vi "关键参数交互.vi"(9 "量程下拉列表":refnum<vi>, 10 "测量模式下拉列表":refnum<vi>, 11 "参数下拉列表":refnum<vi>) -> ()   [LabVIEW 2016]
panel:
  out "x != y? 2":T1
  out "x != y?":T1
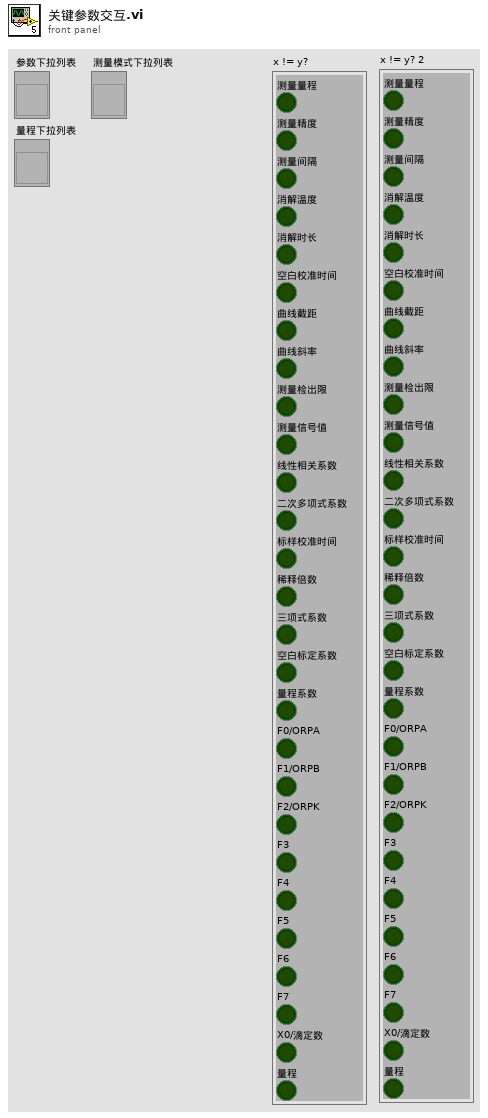
[diagram p1: front panel]
types:
  T1 = cluster{"测量量程":bool, "测量精度":bool, "测量间隔":bool, "消解温度":bool, "消解时长":bool, "空白校准时间":bool, "曲线截距":bool, "曲线斜率":bool, "测量检出限":bool, "测量信号值":bool, "线性相关系数":bool, "二次多项式系数":bool, "标样校准时间":bool, "稀释倍数":bool, "三项式系数":bool, "空白标定系数":bool, "量程系数":bool, "F0/ORPA":bool, "F1/ORPB":bool, "F2/ORPK":bool, "F3":bool, "F4":bool, "F5":bool, "F6":bool, "F7":bool, "X0/滴定数":bool, "量程":bool}
  T2 = cluster{"chose":string, "公式":cluster{"X^2":dbl, "X":dbl, "b":dbl}}
  T3 = cluster{"测量量程":dbl, "测量精度":dbl, "测量间隔":dbl, "消解温度":dbl, "消解时长":dbl, "空白校准时间":timestamp, "曲线截距":dbl, "曲线斜率":dbl, "测量检出限":dbl, "测量信号值":dbl, "线性相关系数":dbl, "二次多项式系数":dbl, "标样校准时间":timestamp, "稀释倍数":dbl, "三项式系数":dbl, "空白标定系数":dbl, "量程系数":dbl, "F0/ORPA":dbl, "F1/ORPB":dbl, "F2/ORPK":dbl, "F3":dbl, "F4":dbl, "F5":dbl, "F6":dbl, "F7":dbl, "X0/滴定数":dbl, "量程":dbl}
  T4 = cluster{"时间标识":timestamp, "设备":string, "日志信息":string, "流程参数":string}
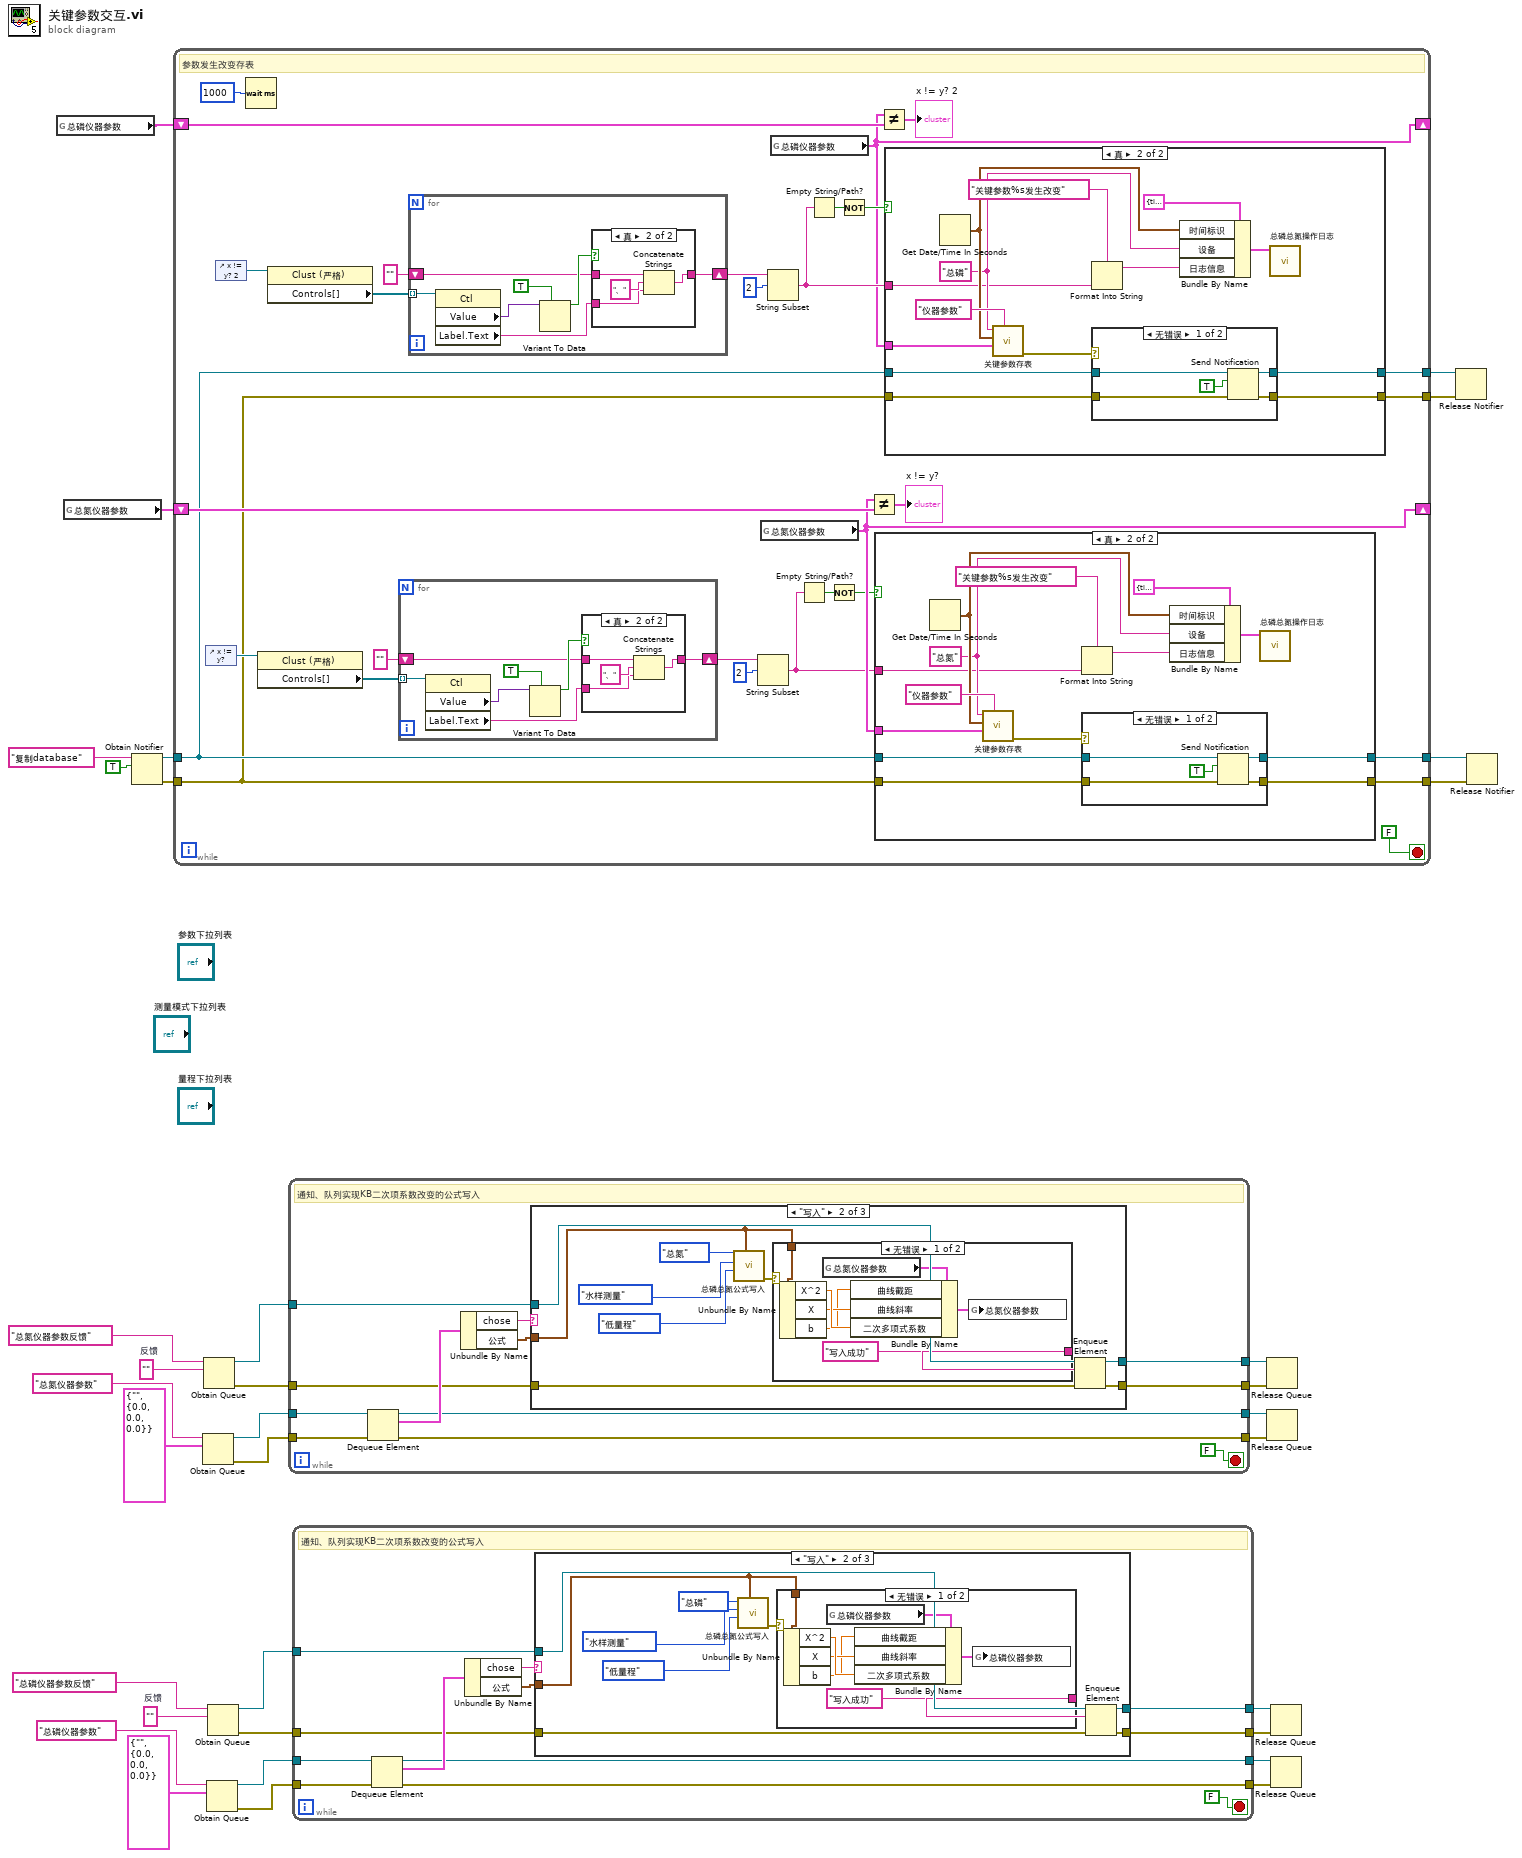
[diagram p0: block diagram]
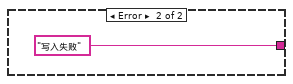
[diagram p3: hidden frame]
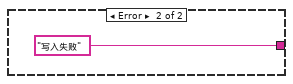
[diagram p6: hidden frame]
diagram:
  w10 = ""  # 反馈
  w27 = ""  # 反馈
  n1 = global read "总磷总氮断电保存全局变量.vi" "总磷仪器参数"() -> (w3:T3)
  n2 = global read "总磷总氮断电保存全局变量.vi" "总氮仪器参数"() -> (w34:T3)
  n3 = Obtain Notifier(name (unnamed)="复制database" ("名称（未命名）"), notification data type=TRUE) -> (notifier out=w19:refnum<notifier>, error out=w18:errorcluster)  [unwired: 2 in, 1 out]
  n4 = while {
    shift-right: [w59] -> _
    shift-left: w34 -> [w62]
    tunnel: w19 -> [w38]
    tunnel: w18 -> [w37]
    tunnel: [w58] -> w17
    tunnel: [w57] -> w16
    shift-right: [w39] -> _
    shift-left: w3 -> [w40]
    tunnel: [w36] -> w2
    tunnel: [w35] -> w1
    stop <- FALSE stop-if-true
    # "参数发生改变存表"
    n5 = control-ref of="x != y?"() -> (w60:refnum<vi>)
    n6 = control-ref of="x != y? 2"() -> (w42:refnum<vi>)
    n7 = Wait (ms)(milliseconds to wait=u32 1000 ("等待时间（毫秒）")) -> ()  [unwired: 1 out]
    n8 = property class="Clust (严格)"(reference=w60) -> ("Controls[]"=w53:refnum<vi>[])  [unwired: 1 in, 2 out]
    n9 = property class="Clust (严格)"(reference=w42) -> ("Controls[]"=w46:refnum<vi>[])  [unwired: 1 in, 2 out]
    n10 = for {
      tunnel: w53 -> [w106] mode=indexing
      shift-right: [w100] -> w55
      shift-left: "" -> [w102]
      n11 = property class="Ctl"(reference=w106) -> ("Value"=w104:variant, "Label.Text"=w101:string)  [unwired: 1 in, 2 out]
      n12 = Variant To Data(type=TRUE, Variant=w104) -> (data=w103:bool)  [unwired: 1 in, 1 out]
      n13 = case shown="真" w103 {
        tunnel: w102 -> [w107 w111]
        tunnel: w101 -> [_ w108]
        tunnel: [w107 w110] -> w100
        frame False {
        }
        frame True {
          n14 = Concatenate Strings(w111, "、", w108) -> (w110:string)
        }
      }
    }
    n15 = for {
      tunnel: w46 -> [w71] mode=indexing
      shift-right: [w65] -> w44
      shift-left: "" -> [w67]
      n16 = property class="Ctl"(reference=w71) -> ("Value"=w69:variant, "Label.Text"=w66:string)  [unwired: 1 in, 2 out]
      n17 = Variant To Data(type=TRUE, Variant=w69) -> (data=w68:bool)  [unwired: 1 in, 1 out]
      n18 = case shown="真" w68 {
        tunnel: w67 -> [w72 w76]
        tunnel: w66 -> [_ w73]
        tunnel: [w72 w75] -> w65
        frame False {
        }
        frame True {
          n19 = Concatenate Strings(w76, "、", w73) -> (w75:string)
        }
      }
    }
    n20 = String Subset(string=w55, offset (0)=2 ("偏移量(0)")) -> (substring=w50:string)  [unwired: 1 in]
    n21 = global read "总磷总氮断电保存全局变量.vi" "总氮仪器参数"() -> (w59:T3)
    n22 = String Subset(string=w44, offset (0)=2 ("偏移量(0)")) -> (substring=w49:string)  [unwired: 1 in]
    n23 = global read "总磷总氮断电保存全局变量.vi" "总磷仪器参数"() -> (w39:T3)
    n24 = Empty String/Path?(string/path=w50) -> (empty?=w52:bool)
    n25 = Empty String/Path?(string/path=w49) -> (empty?=w47:bool)
    n26 = Not(x=w52) -> (.not. x?=w51:bool)
    n27 = Not(x=w47) -> (.not. x?=w48:bool)
    n28 = Not Equal?(x=w59, y=w62) -> (x != y?=→"x != y?":T1)
    n29 = case shown="真" w51 {
      tunnel: w59 -> [_ w126]
      tunnel: w50 -> [_ w120]
      tunnel: w38 -> [w113 w118]
      tunnel: w37 -> [w112 w117]
      tunnel: [w113 w115] -> w58
      tunnel: [w112 w114] -> w57
      frame False {
      }
      frame True {
        w122 = "总氮" ("仪器名称")
        n30 = Get Date/Time In Seconds() -> (seconds since 1Jan1904=w123:timestamp)
        n31 = call "关键参数存表.vi"("table"="仪器参数", "仪器参数"=w126, "datatime"=w123, "仪器名称"=w122) -> ("error out"=w116:errorcluster)  [unwired: 7 in]
        n32 = Format Into String(format string="关键参数%s发生改变" ("格式字符串"), w120) -> (resulting string=w119:string)  [unwired: 2 in, 1 out]
        n33 = case shown="无错误" w116 {
          tunnel: w118 -> [w132 w134]
          tunnel: w117 -> [w131 w133]
          tunnel: [w129 w134] -> w115
          tunnel: [w128 w133] -> w114
          frame No Error {
            n34 = Send Notification(notification=TRUE ("通知"), notifier=w132, error in (no error)=w131) -> (notifier out=w129:refnum<notifier>, error out=w128:errorcluster)
          }
          frame Error {
          }
        }
        n35 = Bundle By Name(cluster=T4 {"时间标识"=timestamp(0 s since 1904-01-01), "设备"="", "日志信息"="", "流程参数"=""} ("data in"), "时间标识"=w123, "设备"=w122, "日志信息"=w119) -> (w124:T4)
        n36 = call "总磷总氮操作日志.vi"("data in"=w124) -> ()  [unwired: 11 in]
      }
    }
    n37 = Not Equal?(x=w39, y=w40) -> (x != y?=→"x != y? 2":T1)
    n38 = case shown="真" w48 {
      tunnel: w39 -> [_ w91]
      tunnel: w49 -> [_ w85]
      tunnel: w38 -> [w78 w83]
      tunnel: w37 -> [w77 w82]
      tunnel: [w78 w80] -> w36
      tunnel: [w77 w79] -> w35
      frame False {
      }
      frame True {
        w87 = "总磷" ("仪器名称")
        n39 = Get Date/Time In Seconds() -> (seconds since 1Jan1904=w88:timestamp)
        n40 = call "关键参数存表.vi"("table"="仪器参数", "仪器参数"=w91, "datatime"=w88, "仪器名称"=w87) -> ("error out"=w81:errorcluster)  [unwired: 7 in]
        n41 = Format Into String(format string="关键参数%s发生改变" ("格式字符串"), w85) -> (resulting string=w84:string)  [unwired: 2 in, 1 out]
        n42 = case shown="无错误" w81 {
          tunnel: w83 -> [w97 w99]
          tunnel: w82 -> [w96 w98]
          tunnel: [w94 w99] -> w80
          tunnel: [w93 w98] -> w79
          frame No Error {
            n43 = Send Notification(notification=TRUE ("通知"), notifier=w97, error in (no error)=w96) -> (notifier out=w94:refnum<notifier>, error out=w93:errorcluster)
          }
          frame Error {
          }
        }
        n44 = Bundle By Name(cluster=T4 {"时间标识"=timestamp(0 s since 1904-01-01), "设备"="", "日志信息"="", "流程参数"=""} ("data in"), "时间标识"=w88, "设备"=w87, "日志信息"=w84) -> (w89:T4)
        n45 = call "总磷总氮操作日志.vi"("data in"=w89) -> ()  [unwired: 11 in]
      }
    }
  }
  n46 = Obtain Queue(name (unnamed)="总氮仪器参数" ("名称（未命名）"), element data type=T2 {"chose"="", "公式"={"X^2"=0.0, "X"=0.0, "b"=0.0}}) -> (queue out=w23:refnum<queue>, error out=w22:errorcluster)  [unwired: 3 in, 1 out]
  n47 = Obtain Queue(name (unnamed)="总氮仪器参数反馈" ("名称（未命名）"), element data type=w27) -> (queue out=w28:refnum<queue>, error out=w26:errorcluster)  [unwired: 3 in, 1 out]
  n48 = Obtain Queue(name (unnamed)="总磷仪器参数" ("名称（未命名）"), element data type=T2 {"chose"="", "公式"={"X^2"=0.0, "X"=0.0, "b"=0.0}}) -> (queue out=w14:refnum<queue>, error out=w15:errorcluster)  [unwired: 3 in, 1 out]
  n49 = Obtain Queue(name (unnamed)="总磷仪器参数反馈" ("名称（未命名）"), element data type=w10) -> (queue out=w9:refnum<queue>, error out=w11:errorcluster)  [unwired: 3 in, 1 out]
  n50 = while {
    tunnel: w23 -> [w145]
    tunnel: w22 -> [w144]
    tunnel: [w136] -> w31
    tunnel: [w135] -> w30
    tunnel: w28 -> [w140]
    tunnel: w26 -> [w139]
    tunnel: [w138] -> w25
    tunnel: [w137] -> w24
    stop <- FALSE stop-if-true
    # "通知、队列实现KB二次项系数改变的公式写入"
    n51 = Dequeue Element(queue=w145, error in (no error)=w144) -> (queue out=w136:refnum<queue>, element=w143:T2, error out=w135:errorcluster)  [unwired: 1 in, 1 out]
    n52 = Unbundle By Name(w143) -> ("chose"=w142:string, "公式"=w141:cluster{"X^2":dbl, "X":dbl, "b":dbl})
    n53 = case shown="\"写入\"" w142 {
      tunnel: w141 -> [_ w152 _]
      tunnel: w140 -> [w148 w157 w168]
      tunnel: w139 -> [w147 w155 w167]
      tunnel: [w148 w154 w168] -> w138
      tunnel: [w147 w153 w167] -> w137
      frame "假", Default {
      }
      frame "写入" {
        n54 = call "总磷总氮公式写入.vi"("公式"=w152, "量程"=enum16{"低量程", "高量程"}."低量程", "测量模式"=enum16{"水样测量", "零点核查", "跨度核查", "标样核查", "加标回收"}."水样测量", "测量参数"=enum16{"总磷", "总氮"}."总氮") -> ("error out"=w158:errorcluster)  [unwired: 7 in]
        n55 = case shown="无错误" w158 {
          tunnel: ["写入成功" ("消息") "写入失败" ("消息")] -> w156
          tunnel: w152 -> [w162 _]
          frame No Error {
            n56 = Unbundle By Name(w162) -> ("X^2"=w161:dbl, "X"=w160:dbl, "b"=w159:dbl)
            n57 = global read "总磷总氮断电保存全局变量.vi" "总氮仪器参数"() -> (w163:T3)
            n58 = Bundle By Name(cluster=w163, "曲线截距"=w159, "曲线斜率"=w160, "二次多项式系数"=w161) -> (w164:T3)
            n59 = global write "总磷总氮断电保存全局变量.vi" "总氮仪器参数"(w164) -> ()
          }
          frame Error {
          }
        }
        n60 = Enqueue Element(queue=w157, element=w156, error in (no error)=w155) -> (queue out=w154:refnum<queue>, error out=w153:errorcluster)  [unwired: 1 in, 1 out]
      }
      frame "读取" {
      }
    }
  }
  n61 = while {
    tunnel: w14 -> [w179]
    tunnel: w15 -> [w178]
    tunnel: [w170] -> w6
    tunnel: [w169] -> w7
    tunnel: w9 -> [w174]
    tunnel: w11 -> [w173]
    tunnel: [w172] -> w12
    tunnel: [w171] -> w13
    stop <- FALSE stop-if-true
    # "通知、队列实现KB二次项系数改变的公式写入"
    n62 = Dequeue Element(queue=w179, error in (no error)=w178) -> (queue out=w170:refnum<queue>, element=w177:T2, error out=w169:errorcluster)  [unwired: 1 in, 1 out]
    n63 = Unbundle By Name(w177) -> ("chose"=w176:string, "公式"=w175:cluster{"X^2":dbl, "X":dbl, "b":dbl})
    n64 = case shown="\"写入\"" w176 {
      tunnel: w175 -> [_ w186 _]
      tunnel: w174 -> [w182 w191 w202]
      tunnel: w173 -> [w181 w189 w201]
      tunnel: [w182 w188 w202] -> w172
      tunnel: [w181 w187 w201] -> w171
      frame "假", Default {
      }
      frame "写入" {
        n65 = call "总磷总氮公式写入.vi"("公式"=w186, "量程"=enum16{"低量程", "高量程"}."低量程", "测量模式"=enum16{"水样测量", "零点核查", "跨度核查", "标样核查", "加标回收"}."水样测量", "测量参数"=enum16{"总磷", "总氮"}."总磷") -> ("error out"=w192:errorcluster)  [unwired: 7 in]
        n66 = case shown="无错误" w192 {
          tunnel: ["写入成功" ("消息") "写入失败" ("消息")] -> w190
          tunnel: w186 -> [w196 _]
          frame No Error {
            n67 = Unbundle By Name(w196) -> ("X^2"=w195:dbl, "X"=w194:dbl, "b"=w193:dbl)
            n68 = global read "总磷总氮断电保存全局变量.vi" "总磷仪器参数"() -> (w197:T3)
            n69 = Bundle By Name(cluster=w197, "曲线截距"=w193, "曲线斜率"=w194, "二次多项式系数"=w195) -> (w198:T3)
            n70 = global write "总磷总氮断电保存全局变量.vi" "总磷仪器参数"(w198) -> ()
          }
          frame Error {
          }
        }
        n71 = Enqueue Element(queue=w191, element=w190, error in (no error)=w189) -> (queue out=w188:refnum<queue>, error out=w187:errorcluster)  [unwired: 1 in, 1 out]
      }
      frame "读取" {
      }
    }
  }
  n72 = Release Queue(queue=w25, error in (no error)=w24) -> ()  [unwired: 1 in, 3 out]
  n73 = Release Queue(queue=w31, error in (no error)=w30) -> ()  [unwired: 1 in, 3 out]
  n74 = Release Queue(queue=w12, error in (no error)=w13) -> ()  [unwired: 1 in, 3 out]
  n75 = Release Queue(queue=w6, error in (no error)=w7) -> ()  [unwired: 1 in, 3 out]
  n76 = Release Notifier(notifier=w2, error in (no error)=w1) -> ()  [unwired: 1 in, 3 out]
  n77 = Release Notifier(notifier=w17, error in (no error)=w16) -> ()  [unwired: 1 in, 3 out]
